vi "Wait for Server.vi"(6 "Timeout(5000ms)":i32=5000, 8 "error in (no error)":errorcluster, 11 "TcpRouter-Client in":refnum<class "TcpRouter-Client.lvclass">) -> (0 "error out":errorcluster, 1 "wait(ms)":u32, 2 "Server Ready?":bool, 3 "TcpRouter-Client out":refnum<class "TcpRouter-Client.lvclass">)   [LabVIEW 2020, in "CSM-TCP-Router.lvlib" / "TcpRouter-Client.lvclass"]
uses:
  TcpRouter-Client.lvclass
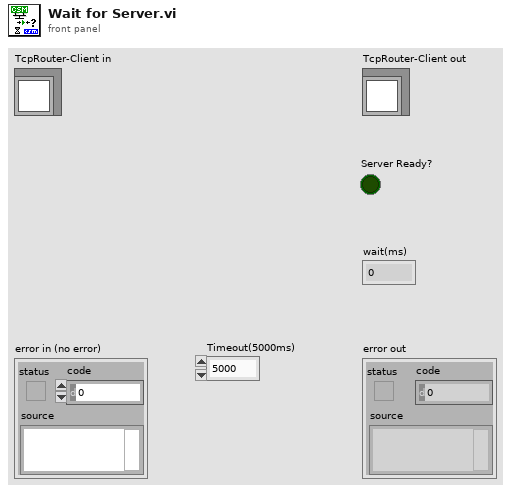
[diagram p1: front panel]
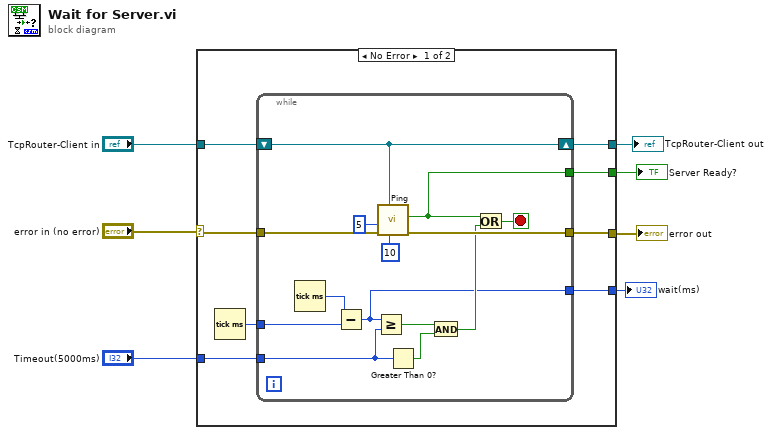
[diagram p0: block diagram]
diagram:
  n1 = case shown="No Error" "error in (no error)" {
    selector: "error in (no error)" -> [w15 w31]
    tunnel: [w12 w31] -> w6
    tunnel: "TcpRouter-Client in" -> [w14 w30]
    tunnel: "Timeout(5000ms)" -> [w10 _]
    tunnel: [w13 _] -> w3
    tunnel: [w9 w30] -> w2
    tunnel: [w8 _] -> w1
    frame No Error {
      n2 = Tick Count (ms)() -> (millisecond timer value=w11:u32)
      n3 = while {
        tunnel: w15 -> [w29]
        tunnel: [w27] -> w13
        tunnel: [w26] -> w12
        tunnel: w11 -> [w25]
        tunnel: w10 -> [w19]
        shift-right: [w18] -> w9
        shift-left: w14 -> [w18]
        tunnel: [w17] -> w8
        stop <- w23 stop-if-true
        n4 = Tick Count (ms)() -> (millisecond timer value=w24:u32)
        n5 = Subtract(x=w24, y=w25) -> (x-y=w17:u32)
        n6 = Greater Or Equal?(x=w17, y=w19) -> (x >= y?=w22:bool)
        n7 = call "Ping.vi"("Response Timeout(100ms)"=10, "TcpRouter-Client in"=w18, "error in (no error)"=w29, "TCP Wait If need connection(ms)"=5) -> ("error out"=w26:errorcluster, "Server Ready?"=w27:bool)  [unwired: 6 in]
        n8 = Greater Than 0?(x=w19) -> (x > 0?=w20:bool)
        n9 = And(x=w22, y=w20) -> (x .and. y?=w21:bool)
        n10 = Or(x=w27, y=w21) -> (x .or. y?=w23:bool)
      }
    }
    frame Error {
    }
  }
  "error out" <- w6
  "Server Ready?" <- w3
  "TcpRouter-Client out" <- w2
  "wait(ms)" <- w1
